vi "punish_check.vi"(1 "input state":T1, 2 "lick":bool, 3 "allow punish":bool) -> (0 "punish":bool)   [LabVIEW 2014]
uses:
  states_def.ctl
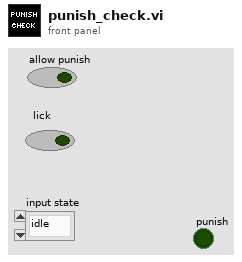
[diagram p1: front panel]
types:
  T1 = typedef "states_def.ctl" = enum16{"idle", "vs before", "vs", "vs after", "delay", "tone before", "tone", "tone after", "cycle end", "reward", "reward refractory", "punish", "punish refractory", "timeout", "exit", "manualwater"}
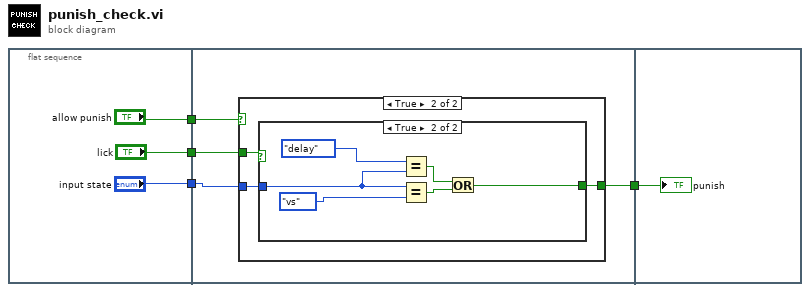
[diagram p0: block diagram]
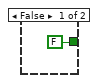
[diagram p2: hidden frame]
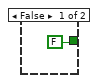
[diagram p3: hidden frame]
diagram:
  n1 = flat-sequence {
    tunnel: ["allow punish"] -> w4
    tunnel: ["input state"] -> w3
    tunnel: ["lick"] -> w2
    tunnel: w4 -> [w11]
    tunnel: w3 -> [w10]
    tunnel: w2 -> [w9]
    tunnel: [w8] -> w1
    tunnel: w1 -> [w23]
    frame #0 {
    }
    frame #1 {
      n2 = case shown="True" w11 {
        tunnel: w10 -> [_ w15]
        tunnel: w9 -> [_ w14]
        tunnel: [FALSE w13] -> w8
        frame False {
        }
        frame True {
          n3 = case shown="True" w14 {
            tunnel: w15 -> [_ w21]
            tunnel: [FALSE w17] -> w13
            frame False {
            }
            frame True {
              n4 = Equal?(x=states_def."delay", y=w21) -> (x = y?=w18:bool)
              n5 = Equal?(x=w21, y=states_def."vs") -> (x = y?=w19:bool)
              n6 = Or(x=w18, y=w19) -> (x .or. y?=w17:bool)
            }
          }
        }
      }
    }
    frame #2 {
      "punish" <- w23
    }
  }
